vi "Create Pattern Script(FSN).vi"(8 "error in (no error)":errorcluster, 11 "FSN":u8) -> (0 "error out":errorcluster, 3 "String":string)   [LabVIEW 2018, in "BML_Frame_Root.lvclass"]
uses:
  BML_Frame_Root.lvclass
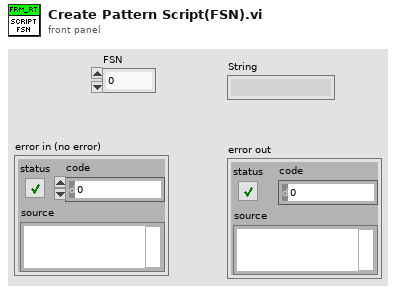
[diagram p1: front panel]
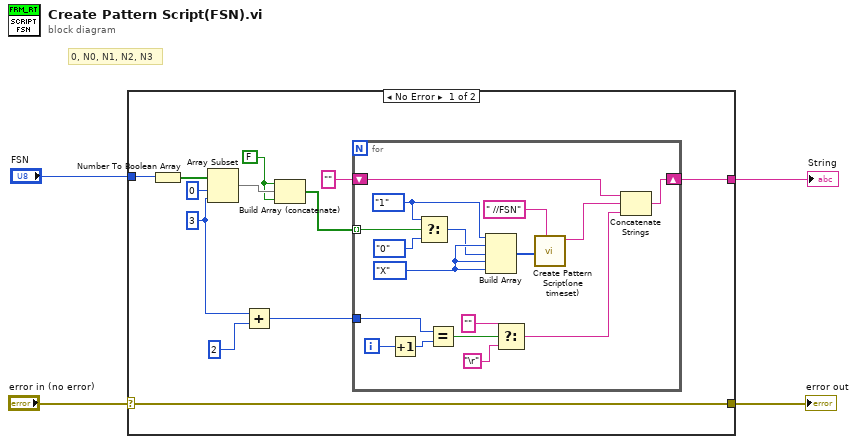
[diagram p0: block diagram]
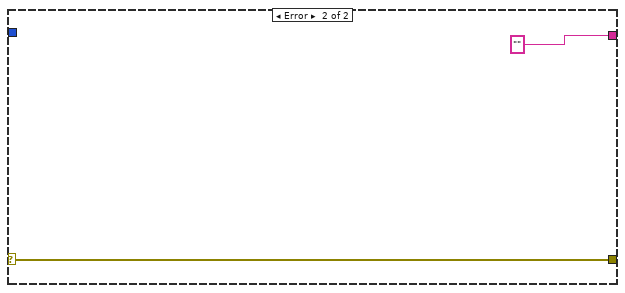
[diagram p2: hidden frame]
diagram:
  # "0, N0, N1, N2, N3"
  n1 = case shown="No Error" "error in (no error)" {
    selector: "error in (no error)" -> [w16 w34]
    tunnel: [w5 ""] -> w3
    tunnel: [w16 w34] -> w2
    tunnel: "FSN" -> [w15 _]
    frame No Error {
      w10 = FALSE
      w8 = 3 ("length")
      n2 = Number To Boolean Array(number=w15) -> (Boolean array=w14:bool[])
      n3 = Array Subset(array=w14, index=0, length=w8) -> (w11:bool[])
      n4 = Add(x=w8, y=2) -> (x+y=w6:i32)
      n5 = Build Array (concatenate)(w10, w11, w10) -> (w9:bool[])
      n6 = for {
        tunnel: w6 -> [w31]
        shift-right: [w25] -> w5
        shift-left: "" -> [w24]
        tunnel: w9 -> [w23] mode=indexing
        i -> [w33]
        w22 = enum16{"0", "1", "L", "H", "X", "V", "D", "M"}."X" ("element")
        w18 = enum16{"0", "1", "L", "H", "X", "V", "D", "M"}."1" ("PinState")
        n7 = Increment(x=w33) -> (x+1=w32:i32)
        n8 = Select(t=w18, s=w23, f=enum16{"0", "1", "L", "H", "X", "V", "D", "M"}."0") -> (s? t:f=w19:enum16{"0", "1", "L", "H", "X", "V", "D", "M"})
        n9 = Equal?(x=w31, y=w32) -> (x = y?=w29:bool)
        n10 = Build Array(w18, w22, w19, w22, w22) -> (w21:enum16{"0", "1", "L", "H", "X", "V", "D", "M"}[])
        n11 = Select(t="", s=w29, f="\r") -> (s? t:f=w26:string)
        n12 = call "Create Pattern Script(one timeset).vi"("Notes"=" //FSN", "PinState"=w21) -> ("string out"=w20:string)  [unwired: 9 in]
        n13 = Concatenate Strings(w24, w20, w26) -> (w25:string)
      }
    }
    frame Error {
    }
  }
  "String" <- w3
  "error out" <- w2
